vi "PID Single.vi"(7 "initialize":bool, 8 "Limits":cluster{"output high":dbl, "output low":dbl}, 9 "PID gains in":T1, 10 "Variable":dbl, 11 "Setpoint":dbl) -> (3 "Out":dbl)   [LabVIEW 2018]
uses:
  <vilib>/ptbypt/NI_PtbyPt.lvlib
panel:
  out "Waveform Chart":dbl[][](graph)
  out "PID Values":dbl[](array[numeric])
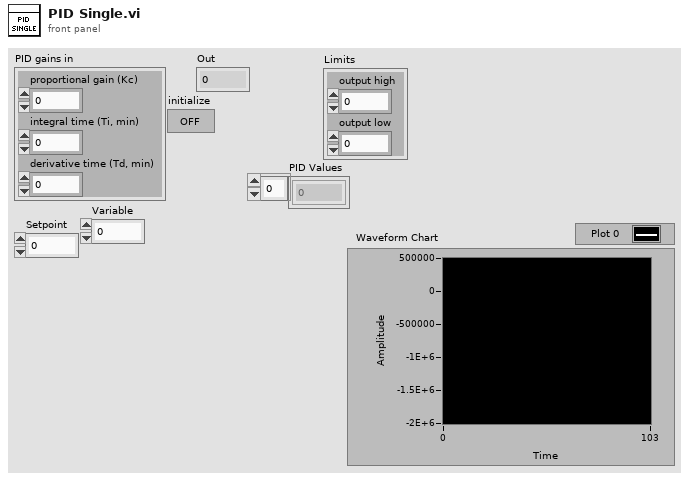
[diagram p1: front panel]
types:
  T1 = cluster{"proportional gain (Kc)":dbl, "integral time (Ti, min)":dbl, "derivative time (Td, min)":dbl}
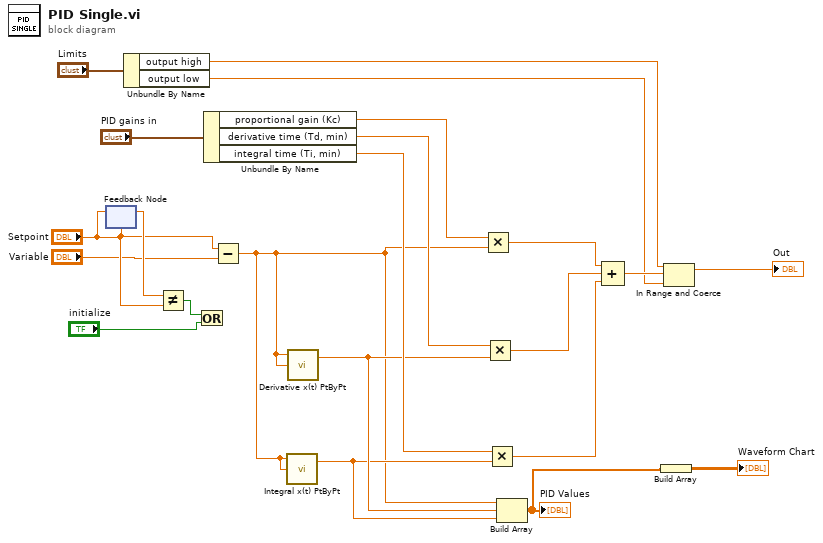
[diagram p0: block diagram]
diagram:
  n1 = feedback-in #1("Setpoint") -> ()
  n2 = feedback #1("Setpoint") -> (w17:dbl)
  n3 = Unbundle By Name("Limits") -> ("output high"=w7:dbl, "output low"=w6:dbl)
  n4 = Not Equal?(x=w17, y="Setpoint") -> (x != y?=w18:bool)
  n5 = Or(x=w18, y="initialize") -> ()  [unwired: 1 out]
  n6 = Unbundle By Name("PID gains in") -> ("proportional gain (Kc)"=w14:dbl, "derivative time (Td, min)"=w13:dbl, "integral time (Ti, min)"=w12:dbl)
  n7 = Subtract(x="Setpoint", y="Variable") -> (x-y=w1:dbl)
  n8 = call <vilib>:"Integral x(t) PtByPt.vi"("initial condition"=w1, "x"=w1) -> ("integral x(t)"=w10:dbl)  [unwired: 2 in, 1 out]
  n9 = call <vilib>:"Derivative x(t) PtByPt.vi"("initial condition"=w1, "x"=w1) -> ("dx/dt"=w11:dbl)  [unwired: 2 in, 1 out]
  n10 = Multiply(x=w14, y=w1) -> (x*y=w8:dbl)
  n11 = Multiply(x=w13, y=w11) -> (x*y=w5:dbl)
  n12 = Multiply(x=w12, y=w10) -> (x*y=w4:dbl)
  n13 = Build Array(w1, w11, w10) -> (w16:dbl[])
  "PID Values" <- w16
  n14 = Compound Arithmetic op=ADD(w8, w5, w4) -> (w9:dbl)
  n15 = Build Array(w16) -> (→"Waveform Chart":dbl[][])
  n16 = In Range and Coerce(upper limit=w7, x=w9, lower limit=w6) -> (coerced(x)=→"Out":dbl)  [unwired: 1 out]
